vi "Write Channel Index.vi"(8 "error in (no error)":errorcluster, 10 "Channel Index":i32, 11 "Digital Toggle Single Msg in":refnum<class "Digital Toggle Single Msg.lvclass">) -> (0 "error out":errorcluster, 3 "Digital Toggle Single Msg out":refnum<class "Digital Toggle Single Msg.lvclass">)   [LabVIEW 2024, in "DAQmx Actor.lvlib" / "Digital Toggle Single Msg.lvclass"]
uses:
  Digital Toggle Single Msg.lvclass
  Digital Toggle Single Msg.lvclass/Digital Toggle Single Msg.ctl
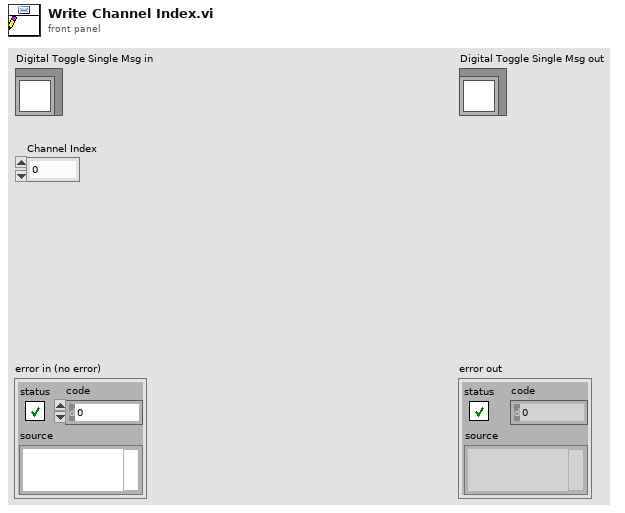
[diagram p1: front panel]
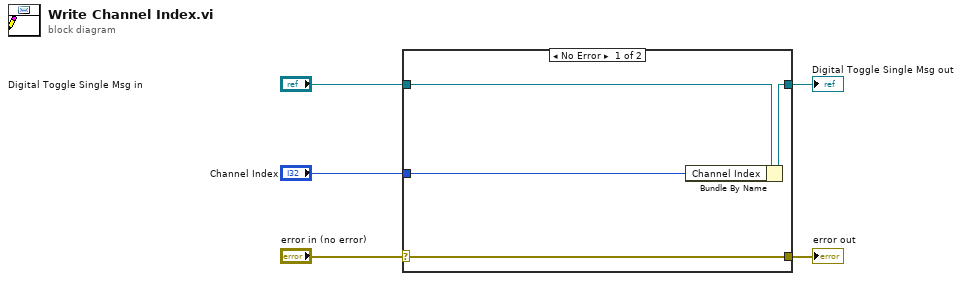
[diagram p0: block diagram]
diagram:
  n1 = case shown="No Error" "error in (no error)" {
    selector: "error in (no error)" -> [w9 w10]
    tunnel: [w9 w10] -> w4
    tunnel: [w7 w11] -> w2
    tunnel: "Digital Toggle Single Msg in" -> [w8 w11]
    tunnel: "Channel Index" -> [w6 _]
    frame No Error {
      n2 = Bundle By Name(cluster=w8, "Channel Index"=w6) -> (w7:refnum<class "Digital Toggle Single Msg.lvclass">)
    }
    frame Error {
    }
  }
  "error out" <- w4
  "Digital Toggle Single Msg out" <- w2
